vi "InitVISA.vi"(0 "object in":refnum<class "DAQ.lvclass">, 2 "ConfigVISA":T1 {"flow control" items=["None"=0, "XON/XOFF"=1, "RTS/CTS"=2, "DTR/DSR"=4]; "stop bits" items=["1.0"=10, "1.5"=15, "2.0"=20]; "parity" items=["None", "Odd", "Even", "Mark", "Space"]; "data bits" min=5 max=8 step=1}, 5 "error in (no error)":errorcluster) -> (14 "object out":refnum<class "DAQ.lvclass">, 19 "error out":errorcluster)   [LabVIEW 2021, in "DAQ.lvclass"]
uses:
  DAQ.lvclass
  ConfigVISA.ctl
  DAQ.lvclass/DAQ.ctl
  <vilib>/Instr/_visa.llb/VISA Configure Serial Port (Instr).vi
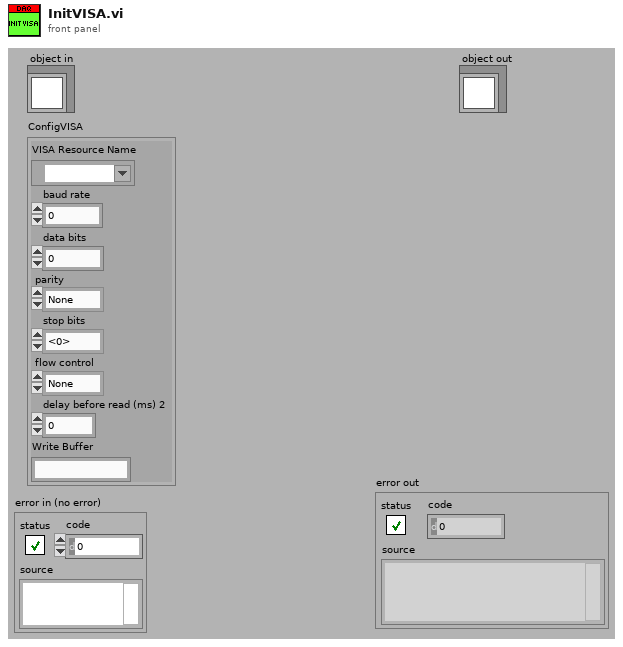
[diagram p1: front panel]
types:
  T1 = typedef "ConfigVISA.ctl" = cluster{"VISA Resource Name":refnum<visa-resource-name>, "baud rate":u32, "data bits":u16, "parity":u16, "stop bits":u16, "flow control":u16, "delay before read (ms) 2":u32, "Write Buffer":string}
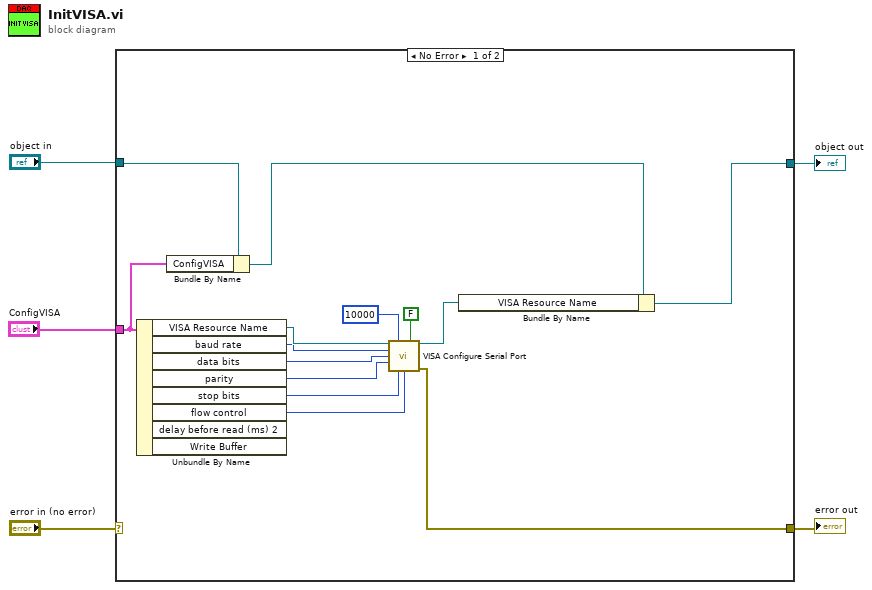
[diagram p0: block diagram]
diagram:
  n1 = case shown="No Error" "error in (no error)" {
    selector: "error in (no error)" -> [_ w21]
    tunnel: [w18 w21] -> w4
    tunnel: [w14 w20] -> w2
    tunnel: "object in" -> [w19 w20]
    tunnel: "ConfigVISA" -> [w13 _]
    frame No Error {
      n2 = Unbundle By Name(w13) -> ("VISA Resource Name"=w12:refnum<visa-resource-name>, "baud rate"=w11:u32, "data bits"=w10:u16, "parity"=w9:u16, "stop bits"=w8:u16, "flow control"=w7:u16)  [unwired: 2 out]
      n3 = Bundle By Name(cluster=w19, "ConfigVISA"=w13) -> (w15:refnum<class "DAQ.lvclass">)
      n4 = call-poly "VISA Configure Serial Port"("VISA resource name"=w12, "timeout (10sec)"=u32 10000, "Enable Termination\nChar (T)"=FALSE ("Enable Termination\nChar (T)"), "baud rate (9600)"=w11, "data bits (8)"=w10, "parity (0:none)"=w9, "stop bits (10: 1 bit)"=w8, "flow control (0:none)"=w7) -> ("VISA resource name out"=w16:refnum<visa-resource-name>, "error out"=w18:errorcluster)  [unwired: 6 in]
      n5 = Bundle By Name(cluster=w15, "VISA Resource Name"=w16) -> (w14:refnum<class "DAQ.lvclass">)
    }
    frame Error {
    }
  }
  "error out" <- w4
  "object out" <- w2
